vi "CodeurRotatif.vi"(8 "codeur":i32) -> (2 "Station Météo":i32)   [LabVIEW 2017]
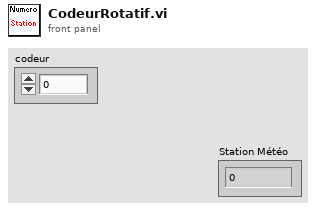
[diagram p1: front panel]
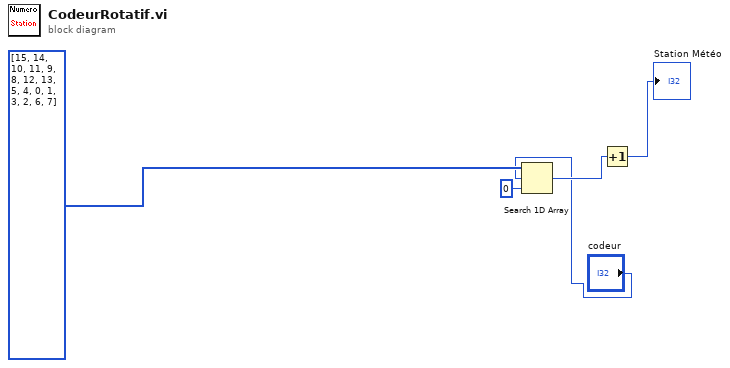
[diagram p0: block diagram]
diagram:
  n1 = Search 1D Array(1D array=i32[] [15, 14, 10, 11, 9, 8, 12, 13, 5, 4, 0, 1, 3, 2, 6, 7], element="codeur", start index (0)=0 ("indice de départ (0)")) -> (index of element=w3:i32)
  n2 = Increment(x=w3) -> (x+1=→"Station Météo":i32)
